vi "BeadTrackerMain.vi"() -> ()   [LabVIEW 2011]
uses:
  qtrk/QTrkLVBinding/QTrkLocalizationType.ctl
  Main/Typedefs/MeasureConfigType.ctl
  Main/Typedefs/MeasureConfigOutputMode.ctl
  qtrk/QTrkLVBinding/QTrkSettings.ctl
  Main/Typedefs/TrackingConfigType.ctl
  qtrk/QTrkLVBinding/QTrkZCommandType.ctl
  Main/ExperimentProgram/ExperimentProgramType.ctl
  Main/ExperimentProgram/ExProgCommandType.ctl
  Main/ExperimentProgram/ExProgCommandEnumType.ctl
  Main/Motors/MotorAxisEnum.ctl
  Main/Motors/MotorPosType.ctl
  Main/Typedefs/XYf.ctl
  Main/Motors/MotorPosFlagsType.ctl
  Main/Camera/GenericCameraConfigType.ctl
  <vilib>/vision/Image Controls.llb/IMAQ Image.ctl
  Main/Camera/PixelCalibrationDataType.ctl
  qtrk/QTrkLVBinding/ResultManagerInstance.ctl
  Main/Typedefs/CmdEnum_UserInterfaceCmd.ctl
  Main/Typedefs/CmdEnum_CameraFrameType.ctl
  Main/GlobalVariables.vi
  Main/Tracking/SemaphoreResultManager.vi
  <vilib>/vision/NI_Vision_Development_Module.lvlib
panel:
  out "Corrected Image buffer":T1
  out "Buffer Image":T1
  in  "Default measure config":T2={"Bead locations"=[{"X"=0, "Y"=0}], "ROI"=80, "Experiment base path"=path "", "Image output subdir"="images", "Output mode"=enum."Track", "Traces output subdir"="traces", "QTrk Settings"={"Image width"=100, "Image height"=100, "Number of threads (CPU based)"=-1, "CUDA Device"=-2, "COM Background correction factor"=0.0, "ZLUT MinRadius"=2.0, "ZLUT Radial sample density"=2.0, "ZLUT Angular sample density"=0.7, "ZLUT ROI Coverage"=1.0, "QI Iterations"=5, "QI MinRadius"=2.0, "QI Radial sample density"=2.0, "QI Angular sample density"=0.7, "QI ROI Coverage"=1.0, "QI Angular Step \nIteration Factor"=1.2, "XCOR Profile Length"=1, "XCOR Profile Width"=128, "XCOR Iterations"=32, "Gaussian 2D Fit Iterations"=2, "Gaussian 2D Sigma (pixels)"=3.0, "Downsample"=0}, "Tracking Config"={"Number of steps"=100, "ZLUT stepsize (um)"=0.05, "Z correction factor"=0.88, "Start piezo Z (um)"=0.0, "Pixel size (nm)"=146.0, "2D Localization Type"=enum."Quadrant Interpolation", "Z Command (None)"=enum."ComputeZ", "Z Piezo scale"=FALSE, "ZLUT Building\nimages per frame"=0, "ZLUT Bias correction planes"=1}, "Experiment Name"="test", "Program"={"Commands"=[], "Motor Axis accuracy conditions"={"Magnet Z"=0.0, "Magnet rotation"=0.0, "Camera"={"X"=0.0, "Y"=0.0}, "Piezo XY"={"X"=0.0, "Y"=0.0}, "Piezo Z"=0.0}, "Axis flags"={"Magnet Z"=FALSE, "Magnet rotation"=FALSE, "Camera"={"X"=FALSE, "Y"=FALSE}, "Piezo XY"={"X"=FALSE, "Y"=FALSE}, "Piezo Z"=FALSE}}, "ZLUT"=[], "Camera settings"={"Framerate (Hz)"=60, "Exposure time (us)"=5000, "Image size"={"Width"=1280, "Height"=1024}, "Number of buffers"=30}, "Experiment Script"="", "Max frames in memory"=100000, "Save traces as binary"=FALSE, "Pixel Calibration Gain Image"="camera_calib_gain.bin", "Pixel Calibration Offset Image"="camera_calib_offset.bin", "Use pixel calibration images"=FALSE, "Internal camera settings"="", "Trace write interval"=100} {"QTrk Settings"."QI ROI Coverage" format="%_2g"; "QTrk Settings"."QI MinRadius" format="%.2f"; "QTrk Settings"."QI Angular sample density" format="%.3f"; "QTrk Settings"."QI Radial sample density" format="%.2f"; "QTrk Settings"."ZLUT Radial sample density" format="%.2f"; "QTrk Settings"."ZLUT MinRadius" format="%.2f"}
  out "Bead positions":cluster{"X":dbl, "Y":dbl}[](array[cluster])
  in  "Compute fisher accuracy":bool
  out "Number of listeners":i32
  out "Running\nexperiment":bool
  out "Cam loop\nupdate speed":dbl
  in  "UpdateTraces":cluster{"ID":dbl}
  in  "UpdateLUT":cluster{"ID":dbl}
  in  "ImageOrResultViewTab":enum32{"Image", "Traces & LUT", "Message Log"}(tab)
  out "Image mean value":sgl(graph)
  in  "Hardware ROI index":i32
  out "Histogram":u32[](graph)
  out "Image":T1(plugin-control)
  out "Frame#":i32
  out "View update rate\n(!= framerate)":dbl caption="View update rate" format="%#_2f"
  in  "Show image?":bool=TRUE
  in  "Histogram":bool
  out "Minimal Value":sgl
  out "Maximal Value":sgl
  in  "Save image":bool
  in  "Pixel calibration":T16(ring)
  out "LUT minimum\nplane index":i32
  in  "Save LUT image":bool
  out "Bead image":u8[][](graph)
  in  "Start frame for trace display":i32(slide) max=9720 scale=0.0..3265.0
  in  "Reference bead#":i32 max=33
  in  "Subtract reference":bool
  in  "Discard bead":bool
  out "Bead XY":sgl[][](graph)
  in  "Bead index":i32 min=0 max=0
  out "Bead Z":sgl[](graph)
  out "Z Lookup Table":sgl[][](graph)
  in  "Number of frames to display":i32=1000 max=33
  out "Bead validity":dbl
  in  "Auto discard":bool
  in  "Minimum bead validity":dbl=1.0
  out "LUT minimum\nplane difference":dbl
  in  "LUT Inspect":bool
  out "Message Log":i32(listbox)
  out "ZLUT":sgl[][][](array[numeric])
  in  "UpdateUI":cluster{"ID":dbl}
  in  "Tab Control":T17(tab)
  out "Camera settings":variant
  in  "Camera settings":bool
  out "Expected location of beadlist:":path
  in  "Load beadlist":bool
  in  "Save beadlist":bool
  in  "ROI":i32=80
  in  "Select beads":bool
  out "Number of beads":i32
  in  "Reload default settings":bool
  in  "Save default settings":bool
  out "Settings location:":path
  in  "Compute&Show zlut bias 2":bool
  in  "ZLUT Bias correction planes":i32=1
  in  "Show zlut bias":bool
  in  "Images per LUT plane":i32
  out "LUT location":path
  in  "Load ZLUT":bool
  in  "Save ZLUT":bool
  in  "2D Localization Type":T6
  in  "Pixel size (nm)":sgl=0.88
  in  "Set current piezo Z as start Z":bool
  in  "Edit QTrk settings":bool
  in  "ZLUT Start piezo Z":sgl=0.88
  in  "Number of steps":i32
  in  "Step size (um)":sgl
  in  "Z correction factor":sgl=0.88
  in  "Build ZLUT":bool
  in  "Select QTrk DLL":bool
  in  "Use LUT scale for Z":bool=TRUE
  in  "Pixel calibration gain:":path
  in  "Pixel calibration offset:":path
  in  "Use gain/offset \ncorrection?":bool
  out "Mean":dbl format="%0.2f"
  out "Mean":dbl format="%0.2f"
  out "Max":sgl
  out "Min":sgl
  out "Max":sgl
  out "Min":sgl
  out "Gain image size":i32[](array[numeric])
  out "Offset image size":i32[](array[numeric])
  out "Variance":dbl format="%0.2f"
  out "Variance":dbl format="%0.2f"
  in  "stop":bool
  # "(used for commands with string parameters)"
  # "-2: Use all devices\n-1: Use best device"
  # "If the camera is giving multiple ROIs, this allows you to select the one that is displayed"
  # "Discard bead also discards bead results and bead ZLUT"
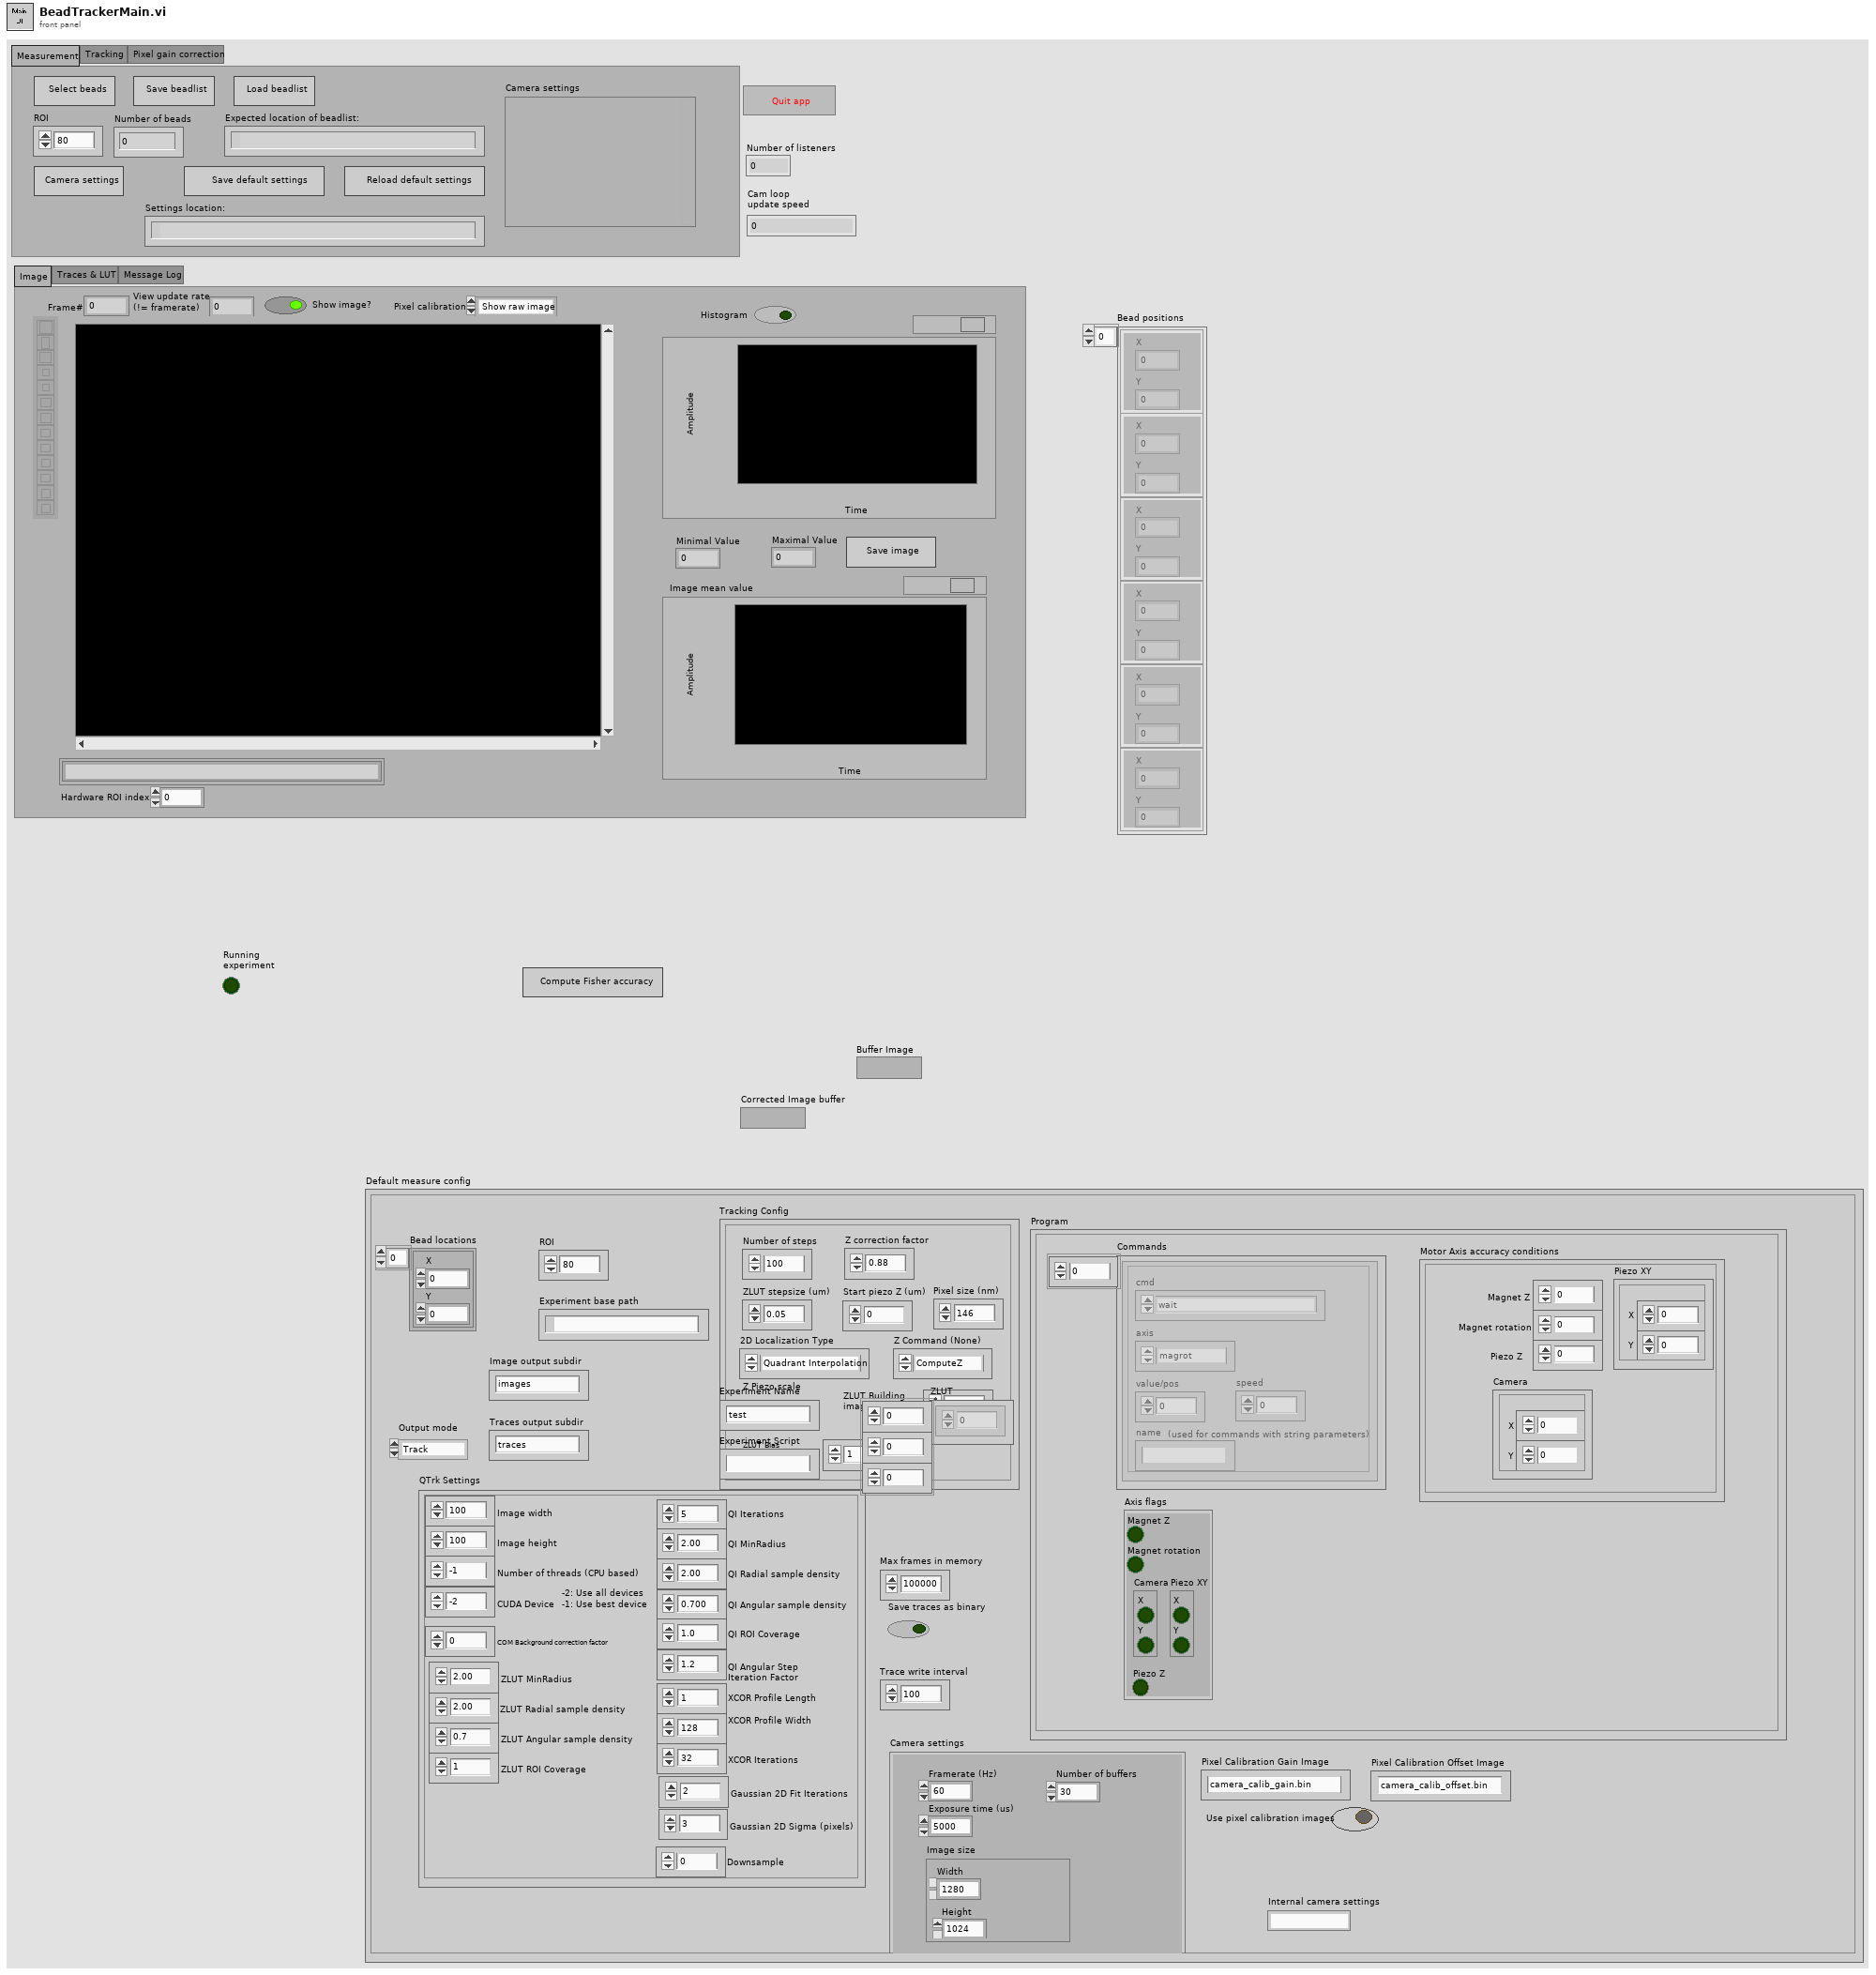
[diagram p1: front panel]
types:
  T1 = typedef "IMAQ Image.ctl" = refnum<image>
  T2 = typedef "MeasureConfigType.ctl" = cluster{"Bead locations":cluster{"X":i32, "Y":i32}[], "ROI":i32, "Experiment base path":path, "Image output subdir":string, "Output mode":T3, "Traces output subdir":string, "QTrk Settings":T4, "Tracking Config":T5, "Experiment Name":string, "Program":T8, "ZLUT":sgl[][][], "Camera settings":T15, "Experiment Script":string, "Max frames in memory":i32, "Save traces as binary":bool, "Pixel Calibration Gain Image":string, "Pixel Calibration Offset Image":string, "Use pixel calibration images":bool, "Internal camera settings":string, "Trace write interval":i32}
  T3 = typedef "MeasureConfigOutputMode.ctl" = enum16{"None", "Track", "SaveImages"}
  T4 = typedef "QTrkSettings.ctl" = cluster{"Image width":i32, "Image height":i32, "Number of threads (CPU based)":i32, "CUDA Device":i32, "COM Background correction factor":sgl, "ZLUT MinRadius":sgl, "ZLUT Radial sample density":sgl, "ZLUT Angular sample density":sgl, "ZLUT ROI Coverage":sgl, "QI Iterations":i32, "QI MinRadius":sgl, "QI Radial sample density":sgl, "QI Angular sample density":sgl, "QI ROI Coverage":sgl, "QI Angular Step \nIteration Factor":sgl, "XCOR Profile Length":i32, "XCOR Profile Width":i32, "XCOR Iterations":i32, "Gaussian 2D Fit Iterations":i32, "Gaussian 2D Sigma (pixels)":sgl, "Downsample":i32}
  T5 = typedef "TrackingConfigType.ctl" = cluster{"Number of steps":i32, "ZLUT stepsize (um)":sgl, "Z correction factor":sgl, "Start piezo Z (um)":sgl, "Pixel size (nm)":sgl, "2D Localization Type":T6, "Z Command (None)":T7, "Z Piezo scale":bool, "ZLUT Building\nimages per frame":i32, "ZLUT Bias correction planes":i32}
  T6 = typedef "QTrkLocalizationType.ctl" = enum16{"Center-of-Mass", "1D Cross-Correlation", "Quadrant Interpolation", "Gaussian 2D MLE", "QI + ZLUTAlign", "ZLUTAlign", "QI + FourierLUT"}
  T7 = typedef "QTrkZCommandType.ctl" = enum16{"Nothing", "ComputeZ", "BuildRadialZLUT", "BuildImageZLUT", "RadialZLUT+ImageZLUT"}
  T8 = typedef "ExperimentProgramType.ctl" = cluster{"Commands":T9[], "Motor Axis accuracy conditions":T12, "Axis flags":T14}
  T9 = typedef "ExProgCommandType.ctl" = cluster{"cmd":T10, "axis":T11, "value/pos":dbl, "speed":dbl, "name":string}
  T10 = typedef "ExProgCommandEnumType.ctl" = enum16{"wait", "move", "event", "idle", "when", "section", "stop"}
  T11 = typedef "MotorAxisEnum.ctl" = enum16{"no axis", "magrot", "magpos", "px", "py", "pz", "camx", "camy"}
  T12 = typedef "MotorPosType.ctl" = cluster{"Magnet Z":dbl, "Magnet rotation":dbl, "Camera":T13, "Piezo XY":T13, "Piezo Z":dbl}
  T13 = typedef "XYf.ctl" = cluster{"X":sgl, "Y":sgl}
  T14 = typedef "MotorPosFlagsType.ctl" = cluster{"Magnet Z":bool, "Magnet rotation":bool, "Camera":cluster{"X":bool, "Y":bool}, "Piezo XY":cluster{"X":bool, "Y":bool}, "Piezo Z":bool}
  T15 = typedef "GenericCameraConfigType.ctl" = cluster{"Framerate (Hz)":i32, "Exposure time (us)":i32, "Image size":cluster{"Width":i32, "Height":i32}, "Number of buffers":i32}
  T16 = enum16{"Show raw image", "Show corrected", "Show offset", "Show gain"}
  T17 = enum32{"Measurement", "Tracking", "Pixel gain correction"}
  T18 = typedef "PixelCalibrationDataType.ctl" = cluster{"Offset image":T1, "Gain image":T1, "Use offset":bool, "Use gain":bool}
  T19 = typedef "CmdEnum_UserInterfaceCmd.ctl" = enum32{"Idle (Use for default)", "ResultTracesUpdated", "MeasureConfigUpdated", "MeasureEnd", "MeasureStart"}
  T20 = typedef "Image Type" = u32
  T21 = typedef "ResultManagerInstance.ctl" = cluster{"InstancePtr":u64}
  T22 = typedef "CameraInstance.ctl" = cluster{"VI refs":T23, "Camera state":variant}
  T23 = typedef "CameraInterface.ctl" = cluster{"Close":T24, "Get/Set generic config":T25, "Grab":T26, "Show Settings Dialog":T27, "AdjustBeadPos":T28, "Save/load camera settings":T29}
  T24 = typedef "CICloseType.ctl" = refnum<vi>
  T25 = typedef "CIGetSetGenericConfig.ctl" = refnum<vi>
  T26 = typedef "CIGrabType.ctl" = refnum<vi>
  T27 = typedef "CISettingsDlg.ctl" = refnum<vi>
  T28 = typedef "CIAdjustBeadPos.ctl" = refnum<vi>
  T29 = typedef "CISaveLoadSettings.ctl" = refnum<vi>
  T30 = typedef "QueueListType.ctl" = cluster{"Motor In":refnum<queue>, "User Interface Image View":refnum<queue>, "User Interface Camera Control":refnum<queue>, "User Interface Event Notifier":refnum<notifier>, "Initialized?":bool, "Experiment Script Event Notifier":refnum<notifier>}
  T31 = cluster{"UpdateUI":refnum<user-event>, "UpdateLUT":refnum<user-event>, "UpdateTraces":refnum<user-event>}
  T32 = typedef "CmdEnum_CameraFrameType.ctl" = enum16{"Full", "HardwareROI", "EndGrabMarker"}
  T33 = typedef "CmdData_NewFrame.ctl" = cluster{"Buffer Image":T1, "Frame #":i32, "Hardware ROI Index":i32, "Timestamp":dbl, "Type":T32}
  T34 = cluster{"histogram":u32[], "Minimal Value":sgl, "Maximal Value":sgl, "Starting Value":sgl, "Interval Width":sgl, "Mean Value":sgl, "Standard  Variation":sgl, "Area (pixels)":i32}
  T35 = enum16{"None", "Normalize", "NormalizeWithoutOffset"}
  T36 = enum16{"big-endian, network order", "native, host order", "little-endian"}
  T37 = enum32{"Invalid", "Standard", "Closed", "Hidden", "Minimized", "Maximized"}
  T38 = typedef "ResultManagerConfig.ctl" = cluster{"Number of beads":i32, "Number of frame info columns":i32, "Result scaling":T39, "Result offset":T39, "Write Interval":i32, "Max frames in memory":i32, "Binary output (1/0)":i8}
  T39 = typedef "XYZf.ctl" = cluster{"X":sgl, "Y":sgl, "Z":sgl}
  T40 = typedef "MotorStateType.ctl" = cluster{"Enabled?":bool, "Current Position":T12, "Update counter":i32}
  T41 = typedef "UserInterfaceEventType.ctl" = cluster{"Type":T19}
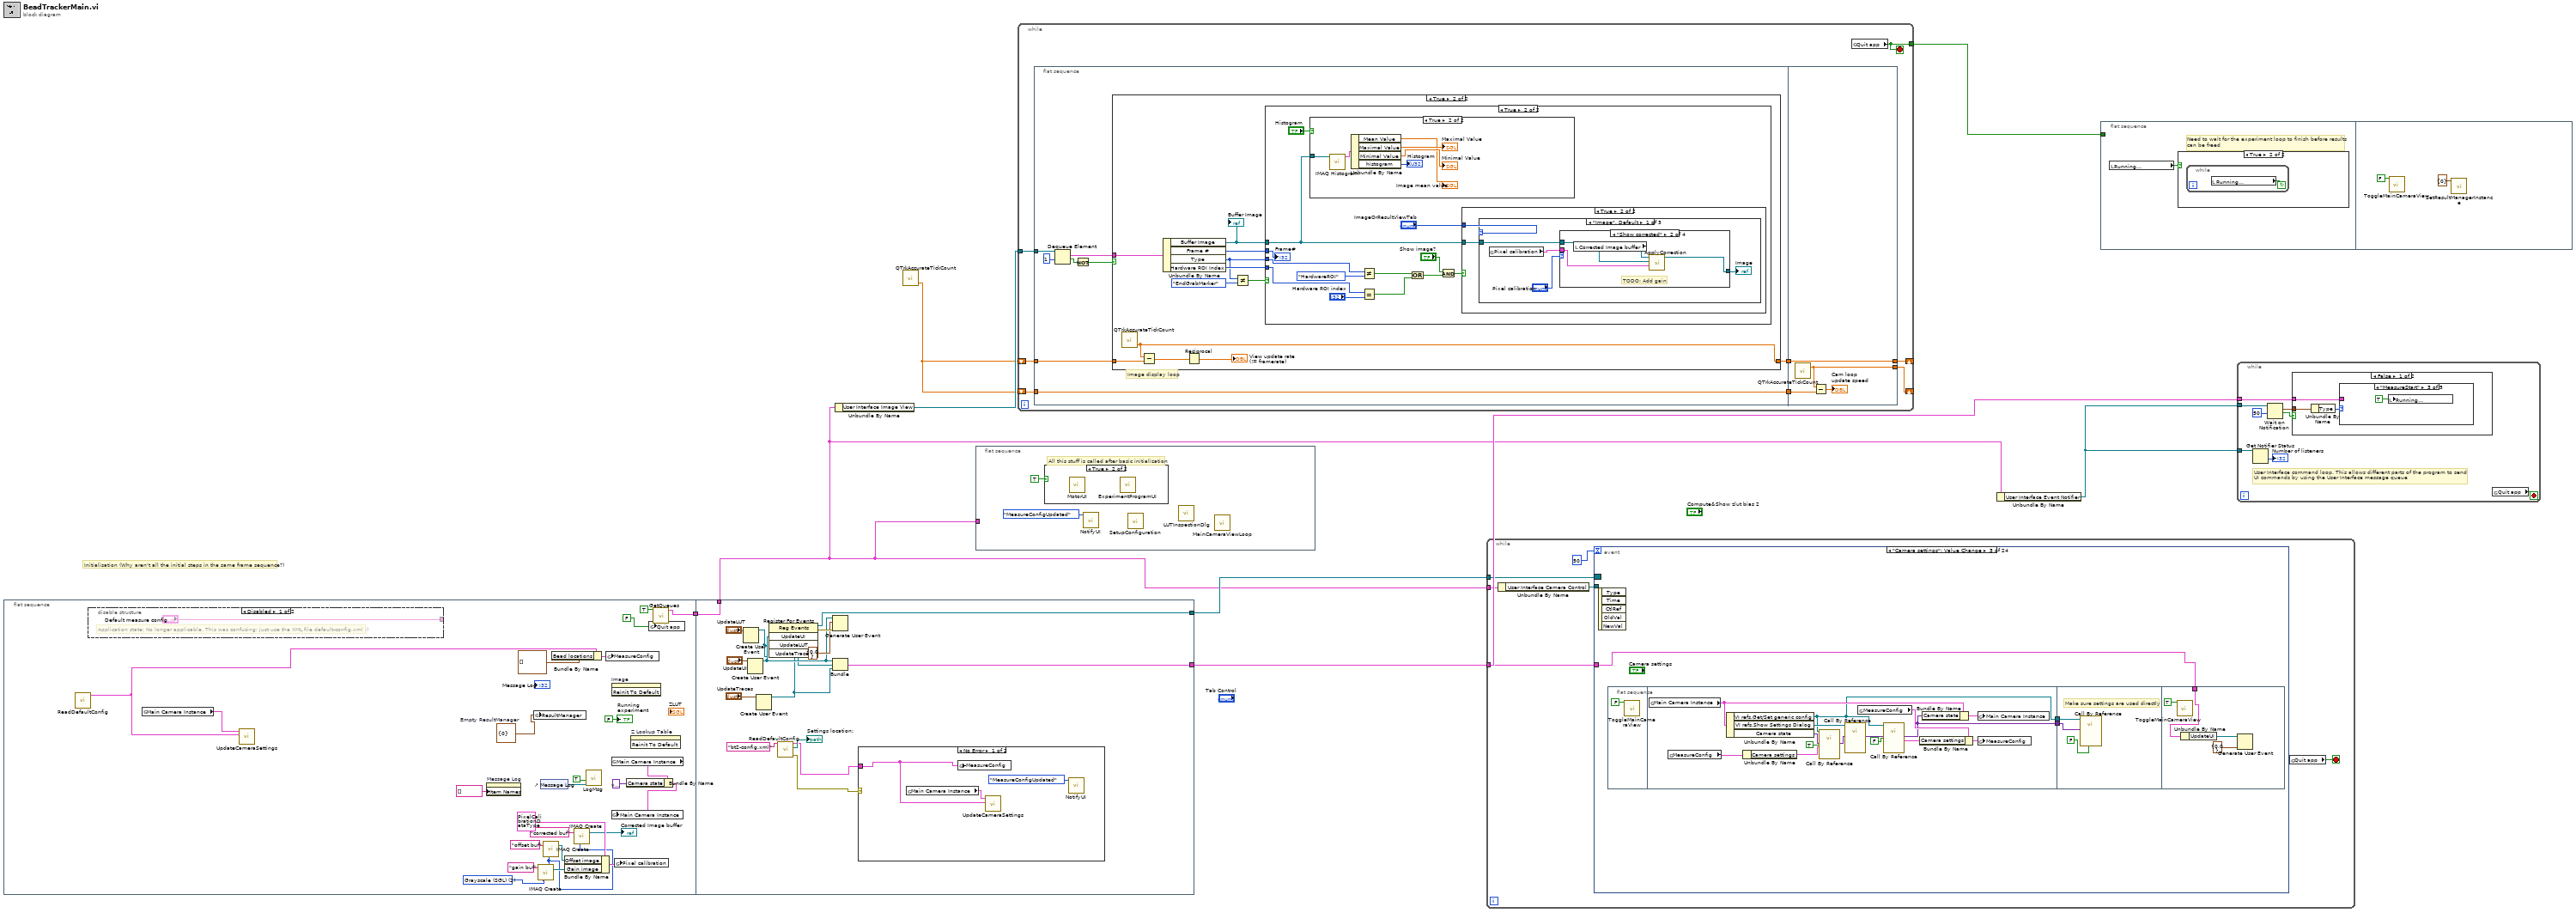
[diagram p0: block diagram]
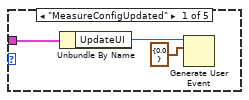
[diagram p3: hidden frame]
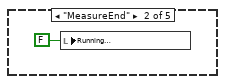
[diagram p4: hidden frame]
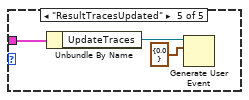
[diagram p6: hidden frame]
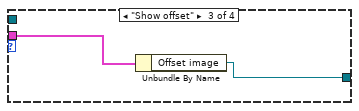
[diagram p16: hidden frame]
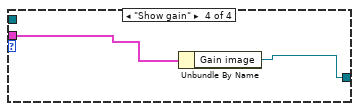
[diagram p17: hidden frame]
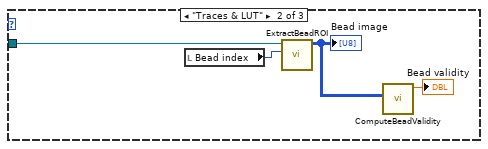
[diagram p18: hidden frame]
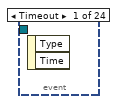
[diagram p20: hidden frame]
diagram:
  # "Initialisation (Why aren't all the initial steps in the same frame sequence?)"
  n1 = flat-sequence {
    tunnel: [w21] -> w2
    tunnel: [w44] -> w8
    tunnel: [w43] -> w4
    tunnel: w2 -> [w38]
    tunnel: [w38] -> w1
    frame #0 {
      w11 = T20 2 items=["Grayscale (U8)", "Grayscale (I16)", "Grayscale (SGL)", "Complex (CSG)", "RGB (U32)", "HSL (U32)", "RGB (U64)", "Grayscale (U16)"] ("Image Type")
      w20 = T21 {"InstancePtr"=0}  # Empty ResultManager
      n2 = call "ReadDefaultConfig.vi"() -> ("config"=w10:T2)  [unwired: 9 in, 2 out]
      n3 = disable-structure shown="Disabled" {
        disable-tunnel: ["Default measure config" _] -> _
        frame Disabled {
          # "Application state: No longer applicable. This was confusing; just use the XML file default-config.xml :)"
        }
        frame Enabled {
        }
      }
      n4 = global read "GlobalVariables.vi" "Main Camera Instance"() -> (w9:T22)
      n5 = call "UpdateCameraSettings.vi"("config"=w10, "Main Camera Instance"=w9) -> ()  [unwired: 10 in]
      n6 = property on="Message Log" class="LstBox (strict)"("Item Names"=string[] []) -> ()  [unwired: 2 in, 2 out]
      n7 = global write "SemaphoreResultManager.vi" "ResultManager"(w20) -> ()
      n8 = call "IMAQ Create"("Image Name"="gain buf", "Image Type"=w11) -> ("New Image"=w15:T1)  [unwired: 3 in, 1 out]
      n9 = control-ref of="Message Log"() -> (w26:refnum<vi>)
      n10 = call "IMAQ Create"("Image Name"="offset buf", "Image Type"=w11) -> ("New Image"=w14:T1)  [unwired: 3 in, 1 out]
      n11 = Bundle By Name(cluster=w10, "Bead locations"=cluster{"X":i32, "Y":i32}[] []) -> (w29:T2)
      n12 = Bundle By Name(cluster=T18 {"Offset image"=refnum, "Gain image"=refnum, "Use offset"=FALSE, "Use gain"=FALSE} ("Pixel calibration"), "Offset image"=w14, "Gain image"=w15) -> (w18:T18)
      n13 = call "IMAQ Create"("Image Name"="corrected buf", "Image Type"=w11) -> ("New Image"=→"Corrected Image buffer":T1)  [unwired: 3 in, 1 out]
      n14 = call "LogMsg.vi"("External listbox\nto add items to"=w26, "Set external listbox"=TRUE) -> ()  [unwired: 10 in]
      n15 = global write "GlobalVariables.vi" "MeasureConfig"(w29) -> ()
      n16 = invoke on="Image" class="ImageControl" method="Reinit To Default"() -> ()  [unwired: 3 in, 3 out]
      n17 = global read "GlobalVariables.vi" "Main Camera Instance"() -> (w24:T22)
      n18 = global write "GlobalVariables.vi" "Pixel calibration"(w18) -> ()
      n19 = Bundle By Name(cluster=w24, "Camera state"=variant ("Variant")) -> (w22:T22)
      n20 = global write "GlobalVariables.vi" "Main Camera Instance"(w22) -> ()
      n21 = invoke on="Z Lookup Table" class="IntGraph (strict)" method="Reinit To Default"() -> ()  [unwired: 3 in, 3 out]
      n22 = global write "GlobalVariables.vi" "Quit app"(FALSE ("Quit app")) -> ()
      n23 = call "GetQueues.vi"("create new? (F)"=TRUE ("create new?")) -> ("Queue List"=w21:T30)  [unwired: 9 in, 1 out]
      "Running\nexperiment" <- FALSE ("Running\nexperiment")
    }
    frame #1 {
      n24 = Create User Event(user event datatype="UpdateLUT") -> (user event=w41:refnum<user-event>)  [unwired: 1 in, 1 out]
      n25 = Create User Event(user event datatype="UpdateUI") -> (user event=w46:refnum<user-event>)  [unwired: 1 in, 1 out]
      n26 = Create User Event(user event datatype="UpdateTraces") -> (user event=w39:refnum<user-event>)  [unwired: 1 in, 1 out]
      n27 = register-events(w46, w41, w39) -> (reference out=w44:refnum<event-registration>, error out=w48:errorcluster)  [unwired: 2 in]
      n28 = call "ReadDefaultConfig.vi"("File"="bt2-config.xml" ("name or relative path")) -> ("error out"=w34:errorcluster, "path"=→"Settings location:":path, "config"=w35:T2)  [unwired: 8 in]
      n29 = Generate User Event(user event=w46, event data cluster=cluster{"ID":dbl} {"ID"=0.0} ("event data"), error in=w48) -> ()  [unwired: 2 out]
      n30 = Bundle("UpdateUI"=w46, "UpdateLUT"=w41, "UpdateTraces"=w39) -> (w43:T31)  [unwired: 1 in]
      n31 = case shown="No Error" w34 {
        tunnel: w35 -> [w49 _]
        frame No Error {
          n32 = global read "GlobalVariables.vi" "Main Camera Instance"() -> (w50:T22)
          n33 = global write "GlobalVariables.vi" "MeasureConfig"(w49) -> ()
          n34 = call "UpdateCameraSettings.vi"("config"=w49, "Main Camera Instance"=w50) -> ()  [unwired: 10 in]
          n35 = call "NotifyUI.vi"("User Interface Commands"=CmdEnum_UserInterfaceCmd."MeasureConfigUpdated") -> ()  [unwired: 11 in]
        }
        frame Error {
        }
      }
    }
  }
  n36 = Unbundle By Name(w1) -> ("User Interface Image View"=w7:refnum<queue>)
  n37 = call "QTrkAccurateTickCount.vi"() -> ("seconds"=w6:dbl)  [unwired: 2 in, 1 out]
  n38 = flat-sequence {
    tunnel: w1 -> [_]
    frame #0 {
      # "All this stuff is called after basic initialization"
      n39 = case shown="True" TRUE {
        frame False {
        }
        frame True {
          n40 = call "MotorUI.vi"() -> ()  [unwired: 12 in]
          n41 = call "ExperimentProgramUI.vi"() -> ()  [unwired: 12 in]
        }
      }
      n42 = call "NotifyUI.vi"("User Interface Commands"=CmdEnum_UserInterfaceCmd."MeasureConfigUpdated") -> ()  [unwired: 11 in]
      n43 = call "SetupConfiguration.vi"() -> ()  [unwired: 12 in]
      n44 = call "LUTInspectionDlg.vi"() -> ()  [unwired: 12 in]
      n45 = call "MainCameraViewLoop.vi"() -> ()  [unwired: 12 in]
    }
  }
  n46 = while {
    tunnel: w7 -> [w61]
    shift-right: [w59] -> _
    shift-left: w6 -> [w60]
    shift-right: [w55] -> _
    shift-left: w6 -> [w56]
    tunnel: [w54] -> w5
    stop <- w54 stop-if-true
    n47 = flat-sequence {
      tunnel: [w69] -> w58
      tunnel: w61 -> [w64]
      tunnel: [w62] -> w57
      tunnel: w56 -> [w69]
      tunnel: w60 -> [w63]
      tunnel: w58 -> [w123]
      tunnel: [w121] -> w59
      tunnel: w57 -> [w121]
      tunnel: [w120] -> w55
      frame #0 {
        # "Image display loop"
        n48 = Dequeue Element(queue=w64, timeout in ms (-1)=1) -> (element=w65:T33, timed out?=w67:bool)  [unwired: 1 in, 2 out]
        n49 = Not(x=w67) -> (.not. x?=w66:bool)
        n50 = case shown="True" w66 {
          tunnel: w65 -> [_ w77]
          tunnel: w63 -> [w70 w81]
          tunnel: [w70 w80] -> w62
          frame False {
          }
          frame True {
            n51 = call "QTrkAccurateTickCount.vi"() -> ("seconds"=w80:dbl)  [unwired: 2 in, 1 out]
            n52 = Subtract(x=w80, y=w81) -> (x-y=w79:dbl)
            n53 = Unbundle By Name(w77) -> ("Buffer Image"=w76:T1, "Frame #"=w71:i32, "Type"=w74:T32, "Hardware ROI Index"=w75:i32)
            "Buffer Image" <- w76
            n54 = Reciprocal(x=w79) -> (1/x=→"View update rate\n(!= framerate)":dbl)
            n55 = Not Equal?(x=w74, y=CmdEnum_CameraFrameType."EndGrabMarker") -> (x != y?=w72:bool)
            n56 = case shown="True" w72 {
              tunnel: w76 -> [_ w93]
              tunnel: w75 -> [_ w91]
              tunnel: w74 -> [_ w85]
              tunnel: w71 -> [_ w86]
              frame False {
              }
              frame True {
                n57 = case shown="True" "Histogram" {
                  tunnel: w93 -> [_ w100]
                  frame False {
                  }
                  frame True {
                    n58 = call "IMAQ Histogram"("Image"=w100) -> ("Histogram Report"=w99:T34)  [unwired: 9 in, 1 out]
                    n59 = Unbundle By Name(w99) -> ("Mean Value"=→"Image mean value":sgl, "Maximal Value"=→"Maximal Value":sgl, "Minimal Value"=→"Minimal Value":sgl, "histogram"=→"Histogram":u32[])
                  }
                }
                n60 = Not Equal?(x=w85, y=CmdEnum_CameraFrameType."HardwareROI") -> (x != y?=w83:bool)
                n61 = Equal?(x=w91, y="Hardware ROI index") -> (x = y?=w89:bool)
                n62 = Or(x=w83, y=w89) -> (x .or. y?=w88:bool)
                n63 = And(x="Show image?", y=w88) -> (x .and. y?=w87:bool)
                n64 = case shown="True" w87 {
                  tunnel: w93 -> [_ w102]
                  tunnel: "ImageOrResultViewTab" -> [_ w101]
                  frame False {
                  }
                  frame True {
                    n65 = case shown="\"Image\", Default" w101 {
                      tunnel: w102 -> [w104 w119 _]
                      frame "Image", Default {
                        n66 = global read "GlobalVariables.vi" "Pixel calibration"() -> (w103:T18)
                        n67 = case shown="\"Show corrected\"" "Pixel calibration" {
                          tunnel: [w107 w110 w113 w115] -> w106
                          tunnel: w104 -> [w107 w109 _ _]
                          tunnel: w103 -> [_ w111 w112 w114]
                          frame "Show raw image", Default {
                          }
                          frame "Show corrected" {
                            # "TODO: Add gain"
                            n68 = local read "Corrected Image buffer"() -> (w108:T1)
                            n69 = call "ApplyCorrection.vi"("Pixel calibration"=w111, "Buffer Image"=w109, "Camera Image"=w108) -> ("Refnum out"=w110:T1)  [unwired: 8 in]
                          }
                          frame "Show offset" {
                            n70 = Unbundle By Name(w112) -> ("Offset image"=w113:T1)
                          }
                          frame "Show gain" {
                            n71 = Unbundle By Name(w114) -> ("Gain image"=w115:T1)
                          }
                        }
                        "Image" <- w106
                      }
                      frame "Traces & LUT" {
                        n72 = local read "Bead index"() -> (w118:i32)
                        n73 = call "ExtractBeadROI.vi"("Bead index"=w118, "Image"=w119) -> ("Image Pixels (U8)"=w117:u8[][])  [unwired: 9 in]
                        "Bead image" <- w117
                        n74 = call "ComputeBeadValidity.vi"("Image Pixels (U8)"=w117) -> ("Bead validity"=→"Bead validity":dbl)  [unwired: 10 in]
                      }
                      frame "Message Log" {
                      }
                    }
                  }
                }
                "Frame#" <- w86
              }
            }
          }
        }
      }
      frame #1 {
        n75 = call "QTrkAccurateTickCount.vi"() -> ("tick count (ms)"=w120:dbl)  [unwired: 2 in, 1 out]
        n76 = Subtract(x=w120, y=w123) -> (x-y=→"Cam loop\nupdate speed":dbl)
      }
    }
    n77 = global read "GlobalVariables.vi" "Quit app"() -> (w54:bool)
  }
  n78 = while {
    tunnel: w1 -> [w128]
    tunnel: w8 -> [w126]
    tunnel: w4 -> [w125]
    stop <- w124 stop-if-true
    n79 = Unbundle By Name(w128) -> ("User Interface Camera Control"=w127:refnum<queue>)
    n80 = event shown="[2] \"Camera settings\": Value Change" {
      selector: w126 -> [_ _ _ _ _ _ _ _ _ _ _ _ _ _ _ _ _ _ _ _ _ _ _ _]
      dyn-events: _ -> [_ _ _ _ _ _ _ _ _ _ _ _ _ _ _ _ _ _ _ _ _ _ _ _]
      timeout: 50 -> [_ _ _ _ _ _ _ _ _ _ _ _ _ _ _ _ _ _ _ _ _ _ _ _]
      tunnel: w127 -> [_ _ _ _ _ _ _ _ _ _ _ _ _ _ _ _ _ _ _ _ _ _ _ _]
      tunnel: w125 -> [_ _ w133 w159 _ _ _ w237 _ _ _ _ w271 w285 _ _ w299 _ w347 _ _ _ _ w375]
      event Timeout {
        n81 = event-data() -> ()  [unwired: 1 in, 2 out]
      }
      event "stop": Value Change {
        n82 = event-data() -> ()  [unwired: 1 in, 5 out]
        n83 = local read "Running\nexperiment"() -> (w130:bool)
        n84 = case shown="True" w130 {
          frame False {
            n85 = global write "GlobalVariables.vi" "Quit app"(TRUE ("Quit app")) -> ()
          }
          frame True {
            n86 = One Button Dialog(message="Abort experiment first") -> ()  [unwired: 1 in, 1 out]
          }
        }
      }
      event "Camera settings": Value Change {
        n87 = event-data() -> ()  [unwired: 1 in, 5 out]
        n88 = flat-sequence {
          tunnel: [w138] -> w135
          tunnel: [w137] -> w134
          tunnel: w135 -> [w154]
          tunnel: w134 -> [w153]
          tunnel: w133 -> [w156]
          frame #0 {
            n89 = call "ToggleMainCameraView.vi"("Enable? (T)"=FALSE) -> ()  [unwired: 11 in]
          }
          frame #1 {
            n90 = global read "GlobalVariables.vi" "Main Camera Instance"() -> (w150:T22)
            n91 = global read "GlobalVariables.vi" "MeasureConfig"() -> (w142:T2)
            n92 = Unbundle By Name(w150) -> ("VI refs.Get/Set generic config"=w138:T25, "VI refs.Show Settings Dialog"=w151:T27, "Camera state"=w143:variant)
            n93 = Unbundle By Name(w142) -> ("Camera settings"=w141:T15)
            n94 = call-by-ref "?"(reference=w138, "Set? (F)"=TRUE, "GenericCameraConfig"=w141, "Camera state"=w143) -> ("Camera state (out)"=w140:variant)  [unwired: 8 in, 3 out]
            n95 = call-by-ref "?"(reference=w151, "Camera state"=w140) -> ("Camera state (out)"=w148:variant)  [unwired: 11 in, 2 out]
            n96 = global read "GlobalVariables.vi" "MeasureConfig"() -> (w146:T2)
            n97 = call-by-ref "?"(reference=w138, "Set? (F)"=FALSE, "Camera state"=w148) -> ("GenericCameraConfig (out)"=w145:T15, "Camera state (out)"=w137:variant)  [unwired: 9 in, 2 out]
            n98 = Bundle By Name(cluster=w146, "Camera settings"=w145) -> (w144:T2)
            n99 = Bundle By Name(cluster=w150, "Camera state"=w137) -> (w149:T22)
            n100 = global write "GlobalVariables.vi" "Main Camera Instance"(w149) -> ()
            n101 = global write "GlobalVariables.vi" "MeasureConfig"(w144) -> ()
          }
          frame #2 {
            # "Make sure settings are used directly"
            n102 = call-by-ref "?"(reference=w154, "Set? (F)"=FALSE, "Camera state"=w153) -> ()  [unwired: 9 in, 4 out]
          }
          frame #3 {
            n103 = call "ToggleMainCameraView.vi"("Enable? (T)"=TRUE) -> ()  [unwired: 11 in]
            n104 = Unbundle By Name(w156) -> ("UpdateUI"=w157:refnum<user-event>)
            n105 = Generate User Event(user event=w157, event data cluster=cluster{"ID":dbl} {"ID"=0.0} ("event data")) -> ()  [unwired: 1 in, 2 out]
          }
        }
      }
      event "Select beads": Value Change {
        n106 = event-data() -> ()  [unwired: 1 in, 5 out]
        n107 = flat-sequence {
          tunnel: w159 -> [w161]
          frame #0 {
            n108 = local read "Buffer Image"() -> (w160:T1)
            n109 = call "SelectBeads.vi"("Input image"=w160) -> ()  [unwired: 11 in]
          }
          frame #1 {
            n110 = Unbundle By Name(w161) -> ("UpdateUI"=w162:refnum<user-event>)
            n111 = Generate User Event(user event=w162, event data cluster=cluster{"ID":dbl} {"ID"=0.0} ("event data")) -> ()  [unwired: 1 in, 2 out]
          }
        }
      }
      event "ROI", "Number of steps", "Step size (um)", "Z correction factor", "ZLUT Start piezo Z", "Pixel size (nm)", "Use gain/offset \ncorrection?", "Pixel calibration gain:", "Pixel calibration offset:", "Use LUT scale for Z", "Images per LUT plane", "ZLUT Bias correction planes": Value Change {
        n112 = event-data() -> ()  [unwired: 1 in, 5 out]
        n113 = global read "GlobalVariables.vi" "MeasureConfig"() -> (w175:T2)
        n114 = Path To String(path="Pixel calibration gain:") -> (string=w167:string)
        n115 = Path To String(path="Pixel calibration offset:") -> (string=w168:string)
        n116 = Bundle By Name(cluster=w175, "ROI"="ROI", "Tracking Config.Number of steps"="Number of steps", "Tracking Config.ZLUT stepsize (um)"="Step size (um)", "Tracking Config.Z correction factor"="Z correction factor", "Tracking Config.Start piezo Z (um)"="ZLUT Start piezo Z", "Tracking Config.Pixel size (nm)"="Pixel size (nm)", "Tracking Config.2D Localization Type"="2D Localization Type", "Pixel Calibration Gain Image"=w167, "Pixel Calibration Offset Image"=w168, "Use pixel calibration images"="Use gain/offset \ncorrection?", "Tracking Config.Z Piezo scale"="Use LUT scale for Z", "Tracking Config.ZLUT Building\nimages per frame"="Images per LUT plane", "Tracking Config.ZLUT Bias correction planes"="ZLUT Bias correction planes") -> (w176:T2)
        n117 = global write "GlobalVariables.vi" "MeasureConfig"(w176) -> ()
        n118 = call "NotifyUI.vi"("User Interface Commands"=CmdEnum_UserInterfaceCmd."MeasureConfigUpdated") -> ()  [unwired: 11 in]
      }
      event "Save default settings", "Reload default settings": Value Change {
        n119 = event-data() -> ()  [unwired: 1 in, 5 out]
        n120 = local read "Settings location:"() -> (w182:path)
        n121 = case shown="True" "Reload default settings" {
          tunnel: w182 -> [w194 w197]
          frame False {
            n122 = global read "GlobalVariables.vi" "Main Camera Instance"() -> (w191:T22)
            n123 = global read "GlobalVariables.vi" "MeasureConfig"() -> (w187:T2)
            n124 = Unbundle By Name(w191) -> ("VI refs.Save/load camera settings"=w190:T29, "Camera state"=w189:variant)
            n125 = call-by-ref "?"(reference=w190, "Save?"=FALSE, "Camera data"=w189) -> ("Serialized data (out)"=w185:string)  [unwired: 9 in, 3 out]
            n126 = Bundle By Name(cluster=w187, "Internal camera settings"=w185) -> (w186:T2)
            n127 = Bundle By Name(cluster=w186, "ZLUT"=sgl[][][] []) -> (w184:T2)
            n128 = Flatten To XML(anything=w184) -> (xml string=w193:string)
            n129 = Write to Text File(file (use dialog)=w194, text=w193) -> ()  [unwired: 2 in, 3 out]
          }
          frame True {
            n130 = call "ReadDefaultConfig.vi"("path"=w197) -> ("error out"=w196:errorcluster, "config"=w195:T2)  [unwired: 8 in, 1 out]
            n131 = global read "GlobalVariables.vi" "Main Camera Instance"() -> (w198:T22)
            n132 = call "UpdateCameraSettings.vi"("config"=w195, "Main Camera Instance"=w198) -> ()  [unwired: 10 in]
            n133 = case shown="No Error" w196 {
              tunnel: w195 -> [w199 _]
              frame No Error {
                n134 = flat-sequence {
                  tunnel: w199 -> [w200]
                  frame #0 {
                    n135 = global write "GlobalVariables.vi" "MeasureConfig"(w200) -> ()
                  }
                  frame #1 {
                    n136 = call "NotifyUI.vi"("User Interface Commands"=CmdEnum_UserInterfaceCmd."MeasureConfigUpdated") -> ()  [unwired: 11 in]
                  }
                }
              }
              frame Error {
              }
            }
          }
        }
      }
      event User Event; "Reference bead#", "Subtract reference", "Start frame for trace display", "Number of frames to display": Value Change {
        n137 = event-data() -> ()  [unwired: 1 in, 2 out]
        n138 = call "LockUnlockResultManager.vi"() -> ("Valid non-zero instance"=w202:bool, "ResultManager"=w203:T21)  [unwired: 9 in, 1 out]
        n139 = flat-sequence {
          tunnel: w203 -> [w205]
          tunnel: w202 -> [w204]
          frame #0 {
            n140 = case shown="True" w204 {
              tunnel: w205 -> [_ w206]
              frame False {
              }
              frame True {
                w219 = 0 ("lower limit")
                n141 = call "RMGetConfig.vi"("ResultManager"=w206) -> ("config"=w212:T38)  [unwired: 9 in, 1 out]
                n142 = Unbundle By Name(w212) -> ("Number of beads"=w211:i32)
                n143 = Unbundle By Name(w206) -> ("InstancePtr"=w220:u64)
                n144 = Decrement(x=w211) -> (x-1=w218:i32)
                n145 = In Range and Coerce(upper limit=w218, x="Bead index", lower limit=w219) -> (In Range?=w216:bool)  [unwired: 1 out]
                n146 = In Range and Coerce(upper limit=w218, x="Reference bead#", lower limit=w219) -> (In Range?=w210:bool)  [unwired: 1 out]
                n147 = Not Equal To 0?(x=w220) -> (x != 0?=w217:bool)
                n148 = Not(x="Subtract reference") -> (.not. x?=w208:bool)
                n149 = Or(x=w210, y=w208) -> (x .or. y?=w207:bool)
                n150 = Compound Arithmetic op=AND(w217, w216, w207) -> (w215:bool)
                n151 = case shown="True" w215 {
                  tunnel: w206 -> [_ w231]
                  tunnel: "Reference bead#" -> [_ w227]
                  tunnel: "Bead index" -> [_ w226]
                  tunnel: "Subtract reference" -> [_ w225]
                  frame False {
                  }
                  frame True {
                    (unwired) FALSE ("Lock? (T)")
                    n152 = call "RMGetFrameCounters.vi"("ResultManager"=w231) -> ("ResultManager (out)"=w224:T21, "endFrame"=w223:i32)  [unwired: 7 in, 6 out]
                    n153 = Subtract(x=w223, y="Number of frames to display") -> (x-y=w221:i32)
                    n154 = call "GenerateTracePlotData.vi"("Reference bead#"=w227, "ResultManager"=w224, "Subtract reference"=w225, "Number of frames to display"="Number of frames to display", "Start frame for trace display"=w221, "Bead index"=w226) -> ("Bead Z"=→"Bead Z":sgl[], "Bead XY"=w229:sgl[][])  [unwired: 4 in]
                    n155 = Transpose 2D Array(2D array=w229) -> (transposed array=→"Bead XY":sgl[][])
                  }
                }
              }
            }
          }
          frame #1 {
            n156 = call "LockUnlockResultManager.vi"("Lock? (T)"=FALSE) -> ()  [unwired: 8 in, 3 out]
          }
        }
      }
      event "Bead index": Value Change {
        n157 = event-data() -> ()  [unwired: 1 in, 5 out]
        n158 = Unbundle By Name(w237) -> ("UpdateLUT"=w236:refnum<user-event>, "UpdateTraces"=w235:refnum<user-event>)
        n159 = Generate User Event(user event=w236, event data cluster=cluster{"ID":dbl} {"ID"=0.0} ("event data")) -> ()  [unwired: 1 in, 2 out]
        n160 = Generate User Event(user event=w235, event data cluster=cluster{"ID":dbl} {"ID"=0.0} ("event data")) -> ()  [unwired: 1 in, 2 out]
      }
      event "Discard bead": Value Change {
        n161 = event-data() -> ()  [unwired: 1 in, 5 out]
        n162 = local read "Running\nexperiment"() -> (w238:bool)
        n163 = case shown="False" w238 {
          frame False {
            n164 = flat-sequence {
              frame #0 {
                n165 = local read "Reference bead#"() -> (w239:i32)
                n166 = local read "Bead index"() -> (w240:i32)
                n167 = Less?(x=w240, y=w239) -> (x < y?=w241:bool)
                n168 = case shown="True" w241 {
                  tunnel: w239 -> [_ w243]
                  frame False {
                  }
                  frame True {
                    n169 = Decrement(x=w243) -> (x-1=w242:i32)
                    n170 = local write "Reference bead#"(w242) -> ()
                  }
                }
                n171 = call "DiscardBead.vi"("Bead index"=w240) -> ()  [unwired: 11 in]
              }
              frame #1 {
                # "Bead index = min( bead_index, #beads )"
                n172 = global read "GlobalVariables.vi" "MeasureConfig"() -> (w249:T2)
                n173 = Unbundle By Name(w249) -> ("Bead locations"=w248:cluster{"X":i32, "Y":i32}[])
                n174 = Array Size(array=w248) -> (size(s)=w246:i32)
                n175 = local read "Bead index"() -> (w247:i32)
                n176 = Decrement(x=w246) -> (x-1=w245:i32)
                n177 = Max & Min(x=w247, y=w245) -> (min(x,y)=w244:i32)  [unwired: 1 out]
                n178 = local write "Bead index"(w244) -> ()
              }
            }
          }
          frame True {
            n179 = One Button Dialog(message="Can't discard bead while doing experiment") -> ()  [unwired: 1 in, 1 out]
          }
        }
      }
      event "Compute fisher accuracy": Value Change {
        n180 = event-data() -> ()  [unwired: 1 in, 5 out]
        n181 = global read "GlobalVariables.vi" "MeasureConfig"() -> (w251:T2)
        n182 = Unbundle By Name(w251) -> ("ZLUT"=w252:sgl[][][])
        n183 = Empty Array?(array=w252) -> (empty?=w253:bool)
        n184 = case shown="False" w253 {
          tunnel: w251 -> [w256 _]
          frame False {
            n185 = local read "Bead index"() -> (w254:i32)
            n186 = call "ComputeFisherMatrixFromLUT.vi"("Show as dialog?"=TRUE, "MeasureConfig"=w256, "Bead index"=w254) -> ()  [unwired: 8 in, 1 out]
          }
          frame True {
          }
        }
      }
      event "Save image": Value Change {
        n187 = event-data() -> ()  [unwired: 1 in, 5 out]
        n188 = local read "Image"() -> (w261:T1)
        n189 = call "ConvertedFileDialog.vi"("prompt"="Select output filename:") -> ("selected path"=w258:path, "cancelled"=w257:bool)  [unwired: 11 in, 2 out]
        n190 = call "IMAQ ImageToArray"("Image"=w261) -> ("Image Pixels (U8)"=w260:u8[][])  [unwired: 3 in, 4 out]
        n191 = case shown="False" w257 {
          tunnel: w260 -> [w263 _]
          tunnel: w258 -> [w262 _]
          frame False {
            (unwired) 0 ("index")
            n192 = call "WriteArrayAsImage.vi"("Data"=w263, "File Path"=w262) -> ()  [unwired: 10 in]
          }
          frame True {
          }
        }
      }
      event "Save LUT image": Value Change {
        n193 = event-data() -> ()  [unwired: 1 in, 5 out]
        n194 = local read "Z Lookup Table"() -> (w264:sgl[][])
        n195 = call "ConvertedFileDialog.vi"("prompt"="Select output filename:") -> ("selected path"=w265:path, "cancelled"=w266:bool)  [unwired: 11 in, 2 out]
        n196 = case shown="False" w266 {
          tunnel: w265 -> [w270 _]
          tunnel: w264 -> [w269 _]
          frame False {
            n197 = call "WriteArrayAsImage.vi"("Data"=w269, "File Path"=w270, "Normalize Mode"=T35."Normalize") -> ()  [unwired: 9 in]
          }
          frame True {
          }
        }
      }
      event "Build ZLUT": Value Change {
        n198 = event-data() -> ()  [unwired: 1 in, 5 out]
        n199 = flat-sequence {
          tunnel: [w276] -> w272
          tunnel: w272 -> [w282]
          tunnel: w271 -> [w278]
          frame #0 {
            n200 = call "QTrkCheckForDLL.vi"() -> ()  [unwired: 12 in]
            n201 = call "ToggleMainCameraView.vi"("Enable? (T)"=FALSE) -> ()  [unwired: 11 in]
          }
          frame #1 {
            n202 = global read "GlobalVariables.vi" "MeasureConfig"() -> (w275:T2)
            n203 = call "BuildZLUT.vi"("MeasureConfig"=w275) -> ("ZLUT"=w276:sgl[][][])  [unwired: 9 in, 1 out]
            n204 = Bundle By Name(cluster=w275, "ZLUT"=w276) -> (w274:T2)
            n205 = local write "ZLUT"(w276) -> ()
            n206 = global write "GlobalVariables.vi" "MeasureConfig"(w274) -> ()
          }
          frame #2 {
            n207 = Array Size(array=w282) -> (size(s)=w281:i32[])
            n208 = Index Array(array=w281, index=0) -> ()  [unwired: 1 out]
            n209 = Unbundle By Name(w278) -> ("UpdateLUT"=w277:refnum<user-event>)
            n210 = call "ToggleMainCameraView.vi"() -> ()  [unwired: 12 in]
            n211 = Generate User Event(user event=w277, event data cluster=cluster{"ID":dbl} {"ID"=0.0} ("event data")) -> ()  [unwired: 1 in, 2 out]
          }
        }
      }
      event "Set current piezo Z as start Z": Value Change {
        n212 = event-data() -> ()  [unwired: 1 in, 5 out]
        n213 = global read "GlobalVariables.vi" "MotorState"() -> (w289:T40)
        n214 = Unbundle By Name(w289) -> ("Current Position.Piezo Z"=w288:dbl)
        n215 = global read "GlobalVariables.vi" "MeasureConfig"() -> (w284:T2)
        n216 = Unbundle By Name(w285) -> ("UpdateUI"=w287:refnum<user-event>)
        n217 = Generate User Event(user event=w287, event data cluster=cluster{"ID":dbl} {"ID"=0.0} ("event data")) -> ()  [unwired: 1 in, 2 out]
        n218 = Bundle By Name(cluster=w284, "Tracking Config.Start piezo Z (um)"=w288) -> (w283:T2)
        n219 = global write "GlobalVariables.vi" "MeasureConfig"(w283) -> ()
      }
      event "Edit QTrk settings": Value Change {
        n220 = event-data() -> ()  [unwired: 1 in, 5 out]
        n221 = global read "GlobalVariables.vi" "MeasureConfig"() -> (w292:T2)
        n222 = Unbundle By Name(w292) -> ("QTrk Settings"=w294:T4, "ROI"=w290:i32)
        n223 = call "EditQTrkSettingsDialog.vi"("ROI"=w290, "Settings"=w294) -> ("Settings (output)"=w293:T4)  [unwired: 9 in]
        n224 = Bundle By Name(cluster=w292, "QTrk Settings"=w293) -> (w291:T2)
        n225 = global write "GlobalVariables.vi" "MeasureConfig"(w291) -> ()
      }
      event "Save ZLUT": Value Change {
        n226 = event-data() -> ()  [unwired: 1 in, 5 out]
        n227 = global read "GlobalVariables.vi" "MeasureConfig"() -> (w298:T2)
        n228 = Unbundle By Name(w298) -> ("ZLUT"=w296:sgl[][][])
        n229 = call "GetExperimentPaths.vi"("MeasureConfig"=w298) -> ("[base]\\[expname].radialzlut"=w297:path)  [unwired: 6 in, 8 out]
        n230 = Write to Binary File(file (use dialog)=w297, data=w296, 9:T36."little-endian" ("byte order (0:big-endian, network order)")) -> ()  [unwired: 3 in, 3 out]
      }
      event "Load ZLUT": Value Change {
        n231 = event-data() -> ()  [unwired: 1 in, 5 out]
        n232 = global read "GlobalVariables.vi" "MeasureConfig"() -> (w305:T2)
        n233 = call "GetExperimentPaths.vi"("MeasureConfig"=w305) -> ("[base]\\[expname].radialzlut"=w304:path)  [unwired: 6 in, 8 out]
        n234 = Read from Binary File(5:sgl[][][] [] ("ZLUT"), 9:T36."little-endian" ("byte order (0:big-endian, network order)"), 11:w304) -> (2:w300:sgl[][][])  [unwired: 3 in, 3 out]
        n235 = call "CheckZLUTDimensions.vi"("ZLUT"=w300, "MeasureConfig"=w305) -> ("OK?"=w301:bool)  [unwired: 9 in]
        n236 = case shown="True" w301 {
          tunnel: w300 -> [_ w310]
          tunnel: w299 -> [_ w306]
          frame False {
          }
          frame True {
            n237 = Unbundle By Name(w306) -> ("UpdateLUT"=w308:refnum<user-event>)
            n238 = global read "GlobalVariables.vi" "MeasureConfig"() -> (w311:T2)
            n239 = Generate User Event(user event=w308, event data cluster=cluster{"ID":dbl} {"ID"=0.0} ("event data")) -> ()  [unwired: 1 in, 2 out]
            n240 = Bundle By Name(cluster=w311, "ZLUT"=w310) -> (w309:T2)
            n241 = global write "GlobalVariables.vi" "MeasureConfig"(w309) -> ()
          }
        }
      }
      event "Select QTrk DLL": Value Change {
        n242 = event-data() -> ()  [unwired: 1 in, 5 out]
        n243 = local read "Running\nexperiment"() -> (w312:bool)
        n244 = case shown="True" w312 {
          frame False {
            n245 = flat-sequence {
              frame #0 {
                # "The ResultManager can still point to memory in the old DLL"
                n246 = call "SetResultManagerInstance.vi"("ResultManager"=T21 {"InstancePtr"=0}) -> ()  [unwired: 11 in]
              }
              frame #1 {
                n247 = call "QTrkSelectDLLDialog.vi"() -> ()  [unwired: 11 in, 1 out]
              }
            }
          }
          frame True {
            n248 = One Button Dialog(message="Dude, experiments are running") -> ()  [unwired: 1 in, 1 out]
          }
        }
      }
      event User Event {
        n249 = event-data() -> ()  [unwired: 1 in, 4 out]
        n250 = Unbundle By Name(w347) -> ("UpdateLUT"=w346:refnum<user-event>)
        n251 = global read "GlobalVariables.vi" "MeasureConfig"() -> (w341:T2)
        n252 = Unbundle By Name(w341) -> ("Bead locations"=w336:cluster{"X":i32, "Y":i32}[], "ROI"=w357:i32, "Tracking Config"=w356:T5, "Tracking Config.2D Localization Type"=w348:T6, "Camera settings"=→"Camera settings":T15, "Tracking Config.ZLUT Building\nimages per frame"=w334:i32, "Tracking Config.ZLUT Bias correction planes"=w315:i32)  [unwired: 1 out]
        "Bead positions" <- w336
        n253 = Generate User Event(user event=w346, event data cluster=cluster{"ID":dbl} {"ID"=0.0} ("event data")) -> ()  [unwired: 1 in, 2 out]
        n254 = call "GetExperimentPaths.vi"("MeasureConfig"=w341) -> ("[base]\\beadlist.txt"=→"Expected location of beadlist:":path, "[base]\\[expname].radialzlut"=→"LUT location":path)  [unwired: 6 in, 7 out]
        n255 = property on="ROI" class="DigNum (strict)"("Value"=w357) -> ()  [unwired: 2 in, 2 out]
        n256 = Array Size(array=w336) -> (size(s)=w344:i32)
        "Number of beads" <- w344
        n257 = Unbundle By Name(w356) -> ("Number of steps"=w355:i32, "ZLUT stepsize (um)"=w354:sgl, "Z correction factor"=w353:sgl, "Start piezo Z (um)"=w351:sgl, "Pixel size (nm)"=w349:sgl, "Z Piezo scale"=w335:bool)
        n258 = local write "2D Localization Type"(w348) -> ()
        n259 = local write "Images per LUT plane"(w334) -> ()
        n260 = Unbundle By Name(w341) -> ("Pixel Calibration Gain Image"=w338:string, "Pixel Calibration Offset Image"=w339:string, "Use pixel calibration images"=w340:bool)
        n261 = Decrement(x=w344) -> (x-1=w342:i32)
        n262 = property on="Number of steps" class="DigNum (strict)"("Value"=w355) -> ()  [unwired: 2 in, 2 out]
        n263 = property on="Step size (um)" class="DigNum (strict)"("Value"=w354) -> ()  [unwired: 2 in, 2 out]
        n264 = property on="Z correction factor" class="DigNum (strict)"("Value"=w353) -> ()  [unwired: 2 in, 2 out]
        n265 = property on="ZLUT Start piezo Z" class="DigNum (strict)"("Value"=w351) -> ()  [unwired: 2 in, 2 out]
        n266 = property on="Pixel size (nm)" class="DigNum (strict)"("Value"=w349) -> ()  [unwired: 2 in, 2 out]
        n267 = local write "Use LUT scale for Z"(w335) -> ()
        n268 = local write "ZLUT Bias correction planes"(w315) -> ()
        n269 = global read "GlobalVariables.vi" "Pixel calibration"() -> (w331:T18)
        n270 = String To Path(string=w338) -> (path=w333:path)
        n271 = String To Path(string=w339) -> (path=w332:path)
        n272 = local write "Use gain/offset \ncorrection?"(w340) -> ()
        n273 = property on="Bead index" class="DigNum (strict)"("Maximum"=w342, "Minimum"=0.0 ("Data Entry Limits:Minimum")) -> ()  [unwired: 2 in, 2 out]
        n274 = call "UpdatePixelCalibrationImages.vi"("Pixel Calibration Offset Image"=w332, "Pixel Calibration Gain Image"=w333, "Pixel calibration"=w331) -> ("Offset"=w318:sgl[][], "Gain"=w319:sgl[][], "Pixel calibration"=w330:T18)  [unwired: 6 in]
        n275 = global write "GlobalVariables.vi" "Pixel calibration"(w330) -> ()
        n276 = local write "Pixel calibration offset:"(w332) -> ()
        n277 = call "GetPixelCalibrationHistogramReports.vi"("Pixel calibration"=w330) -> ("Gain Histogram Report"=w328:T34, "Offset Histogram Report"=w329:T34)  [unwired: 9 in]
        n278 = Unbundle By Name(w329) -> ("Standard  Variation"=→"Variance":sgl, "Mean Value"=→"Mean":sgl, "Maximal Value"=→"Max":sgl, "Minimal Value"=→"Min":sgl)
        n279 = Unbundle By Name(w328) -> ("Minimal Value"=→"Min":sgl, "Maximal Value"=→"Max":sgl, "Standard  Variation"=→"Variance":sgl, "Mean Value"=→"Mean":sgl)
        n280 = local write "Pixel calibration gain:"(w333) -> ()
        n281 = Array Size(array=w318) -> (size(s)=→"Offset image size":i32[])
        n282 = Array Size(array=w319) -> (size(s)=→"Gain image size":i32[])
      }
      event "Show zlut bias": Value Change {
        n283 = event-data() -> ()  [unwired: 1 in, 5 out]
        n284 = global read "GlobalVariables.vi" "MeasureConfig"() -> (w359:T2)
        n285 = Unbundle By Name(w359) -> ("Tracking Config.ZLUT Bias correction planes"=w358:i32)
        n286 = call "ShowZLUTBias.vi"("Bias planes"=w358) -> ()  [unwired: 11 in]
      }
      event "LUT Inspect": Value Change {
        n287 = event-data() -> ()  [unwired: 1 in, 5 out]
        n288 = vi-ref "LUTInspectionDlg.vi"() -> (w362:refnum<vi>)
        n289 = invoke class="VI (strict)" method="FP.Open"(reference=w362, "Activate"=TRUE ("Activate?"), "State"=T37."Standard") -> ()  [unwired: 2 in, 5 out]
      }
      event "Auto discard": Value Change {
        n290 = event-data() -> ()  [unwired: 1 in, 5 out]
        n291 = local read "Buffer Image"() -> (w364:T1)
        n292 = call "AutoDiscardBeads.vi"("Minimum bead validity"="Minimum bead validity", "Buffer Image"=w364) -> ()  [unwired: 10 in]
      }
      event User Event {
        n293 = event-data() -> ()  [unwired: 1 in, 2 out]
        n294 = global read "GlobalVariables.vi" "MeasureConfig"() -> (w371:T2)
        n295 = Unbundle By Name(w371) -> ("Tracking Config.ZLUT stepsize (um)"=w368:sgl, "Tracking Config.Start piezo Z (um)"=w369:sgl, "ZLUT"=w370:sgl[][][])
        n296 = local read "Bead index"() -> (w372:i32)
        n297 = Index Array(array=w370, index (dim 0)=w372) -> (element=w367:sgl[][])  [unwired: 2 in]
        "Z Lookup Table" <- w367
        n298 = property on="Z Lookup Table" class="IntGraph (strict)"("YScale.Multiplier"=w368, "YScale.Offset"=w369) -> ()  [unwired: 2 in, 2 out]
        n299 = call "LUTPlane2PlaneDist.vi"("ZLUT"=w367) -> ("min index"=→"LUT minimum\nplane index":i32, "min diff"=→"LUT minimum\nplane difference":sgl)  [unwired: 6 in, 3 out]
      }
      event "Save beadlist", "Load beadlist": Value Change {
        n300 = event-data() -> ()  [unwired: 1 in, 5 out]
        n301 = global read "GlobalVariables.vi" "MeasureConfig"() -> (w374:T2)
        n302 = Unbundle By Name(w374) -> ("Bead locations"=w380:cluster{"X":i32, "Y":i32}[])
        n303 = call "GetExperimentPaths.vi"("MeasureConfig"=w374) -> ("[base]\\beadlist.txt"=w379:path)  [unwired: 6 in, 8 out]
        n304 = call "SaveOrLoadBeadlist.vi"("beadlist filename"=w379, "Load beadlist"="Load beadlist", "Bead locations (input)"=w380) -> ("Bead locations (output)"=w378:cluster{"X":i32, "Y":i32}[])  [unwired: 8 in]
        n305 = Unbundle By Name(w375) -> ("UpdateUI"=w377:refnum<user-event>)
        n306 = Bundle By Name(cluster=w374, "Bead locations"=w378) -> (w373:T2)
        n307 = global write "GlobalVariables.vi" "MeasureConfig"(w373) -> ()
        n308 = Generate User Event(user event=w377, event data cluster=cluster{"ID":dbl} {"ID"=0.0} ("event data")) -> ()  [unwired: 1 in, 2 out]
      }
    }
    n309 = global read "GlobalVariables.vi" "Quit app"() -> (w124:bool)
  }
  n310 = Unbundle By Name(w1) -> ("User Interface Event Notifier"=w3:refnum<notifier>)
  n311 = flat-sequence {
    tunnel: w5 -> [_]
    frame #0 {
      # "Need to wait for the experiment loop to finish before results\ncan be freed"
      n312 = local read "Running\nexperiment"() -> (w382:bool)
      n313 = case shown="True" w382 {
        frame False {
        }
        frame True {
          n314 = while {
            stop <- w383 continue-if-true
            n315 = local read "Running\nexperiment"() -> (w383:bool)
          }
        }
      }
    }
    frame #1 {
      n316 = call "ToggleMainCameraView.vi"("Enable? (T)"=FALSE) -> ()  [unwired: 11 in]
      n317 = call "SetResultManagerInstance.vi"("ResultManager"=T21 {"InstancePtr"=0}) -> ()  [unwired: 11 in]
    }
  }
  n318 = while {
    tunnel: w4 -> [w392]
    tunnel: w3 -> [w391]
    tunnel: w3 -> [w388]
    stop <- w393 stop-if-true
    # "User Interface command loop. This allows different parts of the program to send \nUI commands by using the User Interface message queue"
    n319 = Get Notifier Status(notifier=w391) -> (# waiting=→"Number of listeners":i32)  [unwired: 1 in, 4 out]
    n320 = Wait on Notification(notifier=w388, timeout in ms (-1)=50) -> (notification=w386:T41, timed out?=w387:bool)  [unwired: 2 in, 2 out]
    n321 = case shown="False" w387 {
      tunnel: w392 -> [w396 _]
      tunnel: w386 -> [w395 _]
      frame False {
        n322 = Unbundle By Name(w395) -> ("Type"=w394:T19)
        n323 = case shown="\"MeasureStart\"" w394 {
          tunnel: w396 -> [w398 _ _ _ w404]
          frame "MeasureConfigUpdated" {
            n324 = Unbundle By Name(w398) -> ("UpdateUI"=w397:refnum<user-event>)
            n325 = Generate User Event(user event=w397, event data cluster=cluster{"ID":dbl} {"ID"=0.0} ("event data")) -> ()  [unwired: 1 in, 2 out]
          }
          frame "MeasureEnd" {
            n326 = local write "Running\nexperiment"(FALSE ("Running\nexperiment")) -> ()
          }
          frame "MeasureStart" {
            n327 = local write "Running\nexperiment"(TRUE ("Running\nexperiment")) -> ()
          }
          frame Default {
          }
          frame "ResultTracesUpdated" {
            n328 = Unbundle By Name(w404) -> ("UpdateTraces"=w403:refnum<user-event>)
            n329 = Generate User Event(user event=w403, event data cluster=cluster{"ID":dbl} {"ID"=0.0} ("event data")) -> ()  [unwired: 1 in, 2 out]
          }
        }
      }
      frame True {
      }
    }
    n330 = global read "GlobalVariables.vi" "Quit app"() -> (w393:bool)
  }
